vi "json_flatten.vi"(8 "error in (no error)":errorcluster, 11 "json variant":variant) -> (0 "error out":errorcluster, 3 "flattened variant":variant)   [LabVIEW 2011]
doc: "Flatten a nested JSON variant. Keys become dot-delimited."
uses:
  <vilib>/Utility/VariantDataType/Type.ctl
  <vilib>/Utility/VariantDataType/VariantType.lvlib
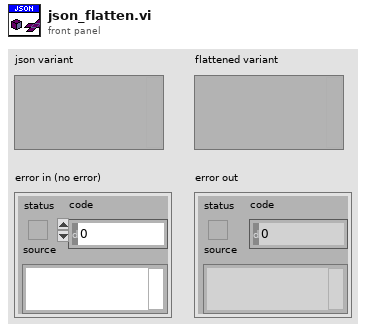
[diagram p1: front panel]
types:
  T1 = typedef "VariantType.lvlib/Type.ctl" = enum8{"Invalid Type", "Void", "I8", "I16", "I32", "I64", "U8", "U16", "U32", "U64", "Single Float", "Double Float", "Extended Float", "Single Complex", "Double Complex", "Extended Complex", "Enum U8", "Enum U16", "Enum U32", "Enum U64", "Single Float With Unit", "Double Float With Unit", "Extended Float With Unit", "Single Complex with Unit", "Double Complex with Unit", "Extended Complex with Unit", "Boolean", "String", "Path", "Picture", "Tag", "Array", "Cluster", "Variant", "LV Variant", "Waveform", "Timestamp", "Digital Waveform", "Digital Data", "ExpressData", "Refnum", "External Data", "VI", "Poly VI", "LabVIEW Class Instance", "Fixed Point"}
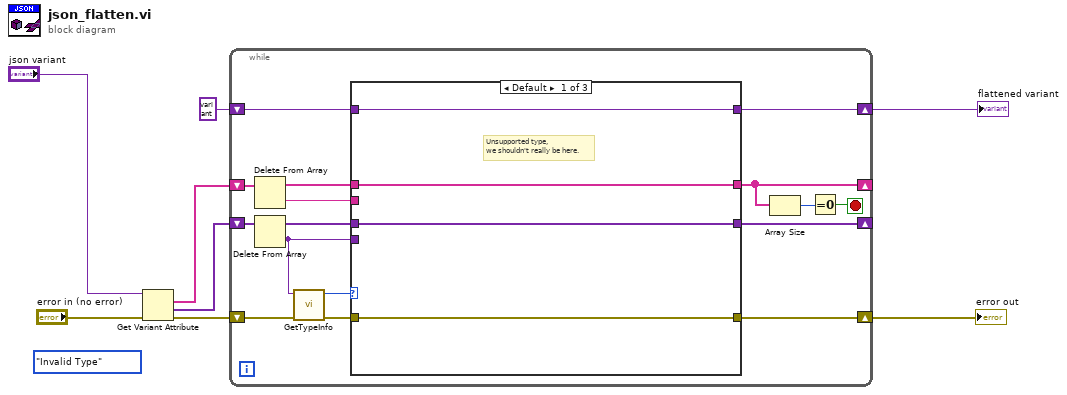
[diagram p0: block diagram]
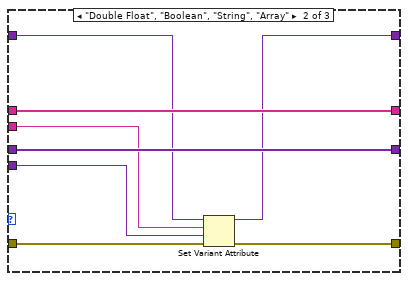
[diagram p2: hidden frame]
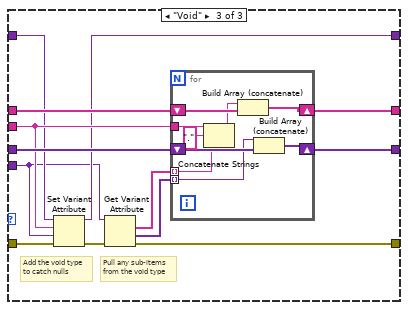
[diagram p3: hidden frame]
diagram:
  (unwired) Type."Invalid Type" ("Type Enum")
  n1 = Get Variant Attribute(Variant="json variant", error in="error in (no error)") -> (names=w5:string[], values=w4:variant[], error out=w6:errorcluster)  [unwired: 2 in, 1 out]
  n2 = while {
    shift-right: [w10] -> w2
    shift-left: variant ("variant") -> [w21]
    shift-right: [w11] -> _
    shift-left: w5 -> [w24]
    shift-right: [w15] -> _
    shift-left: w4 -> [w20]
    shift-right: [w12] -> w1
    shift-left: w6 -> [w19]
    stop <- w22 stop-if-true
    n3 = Delete From Array(array=w24) -> (deleted portion=w13:string, array with subset deleted=w14:string[])  [unwired: 2 in]
    n4 = Delete From Array(array=w20) -> (deleted portion=w9:variant, array with subset deleted=w16:variant[])  [unwired: 2 in]
    n5 = call <vilib>:"GetTypeInfo.vi"("error in (no error)"=w19, "Variant"=w9) -> ("error out"=w18:errorcluster, "Type Enum"=w17:T1)  [unwired: 5 in, 3 out]
    n6 = case shown="Default" w17 {
      tunnel: w21 -> [w26 w31 w41]
      tunnel: w18 -> [w25 w34 w38]
      tunnel: w16 -> [w28 w36 w47]
      tunnel: [w28 w36 w45] -> w15
      tunnel: w14 -> [w27 w35 w48]
      tunnel: w13 -> [_ w32 w42]
      tunnel: [w27 w35 w43] -> w11
      tunnel: [w25 w33 w44] -> w12
      tunnel: [w26 w30 w40] -> w10
      tunnel: w9 -> [_ w29 w39]
      frame Default {
        # "Unsupported type,\nwe shouldn't really be here."
      }
      frame "Double Float", "Boolean", "String", "Array" {
        n7 = Set Variant Attribute(Variant=w31, name=w32, value=w29, error in=w34) -> (Variant out=w30:variant, error out=w33:errorcluster)  [unwired: 1 out]
      }
      frame "Void" {
        # "Pull any sub-items\nfrom the void type"
        # "Add the void type\nto catch nulls"
        n8 = Set Variant Attribute(Variant=w41, name=w42, value=w39, error in=w38) -> (Variant out=w40:variant, error out=w37:errorcluster)  [unwired: 1 out]
        n9 = Get Variant Attribute(Variant=w39, error in=w37) -> (names=w49:string[], values=w46:variant[], error out=w44:errorcluster)  [unwired: 2 in, 1 out]
        n10 = for {
          tunnel: w49 -> [w53] mode=indexing
          shift-right: [w52] -> w43
          shift-left: w48 -> [w58]
          tunnel: w42 -> [w57]
          shift-right: [w50] -> w45
          shift-left: w47 -> [w54]
          tunnel: w46 -> [w51] mode=indexing
          n11 = Concatenate Strings(w57, ".", w53) -> (w55:string)
          n12 = Build Array (concatenate)(w55, w58) -> (w52:string[])
          n13 = Build Array (concatenate)(w51, w54) -> (w50:variant[])
        }
      }
    }
    n14 = Array Size(array=w11) -> (size(s)=w23:i32)
    n15 = Equal To 0?(x=w23) -> (x = 0?=w22:bool)
  }
  "error out" <- w1
  "flattened variant" <- w2
